vi "Day 7.2 - align crabs subs with increasing fuel cost.vi"(11 "input":i32[](array[numeric])) -> (3 "output":i32)   [LabVIEW 2021]
panel:
  out "position":i32
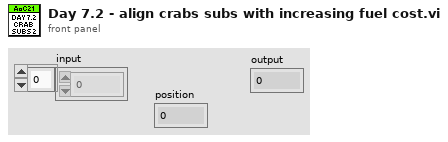
[diagram p1: front panel]
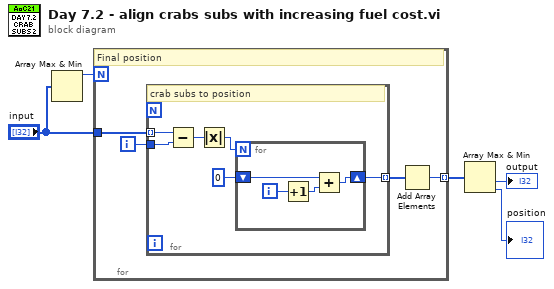
[diagram p0: block diagram]
diagram:
  n1 = Array Max & Min(array="input") -> (max value=w4:i32)  [unwired: 3 out]
  n2 = for {
    N: w4 -> [_]
    tunnel: "input" -> [w9]
    tunnel: [w6] -> w3 mode=indexing
    i -> [w8]
    # "Final position"
    n3 = for {
      tunnel: w8 -> [w14]
      tunnel: w9 -> [w15] mode=indexing
      tunnel: [w10] -> w7 mode=indexing
      # "crab subs to position"
      n4 = Subtract(x=w15, y=w14) -> (x-y=w13:i32)
      n5 = Absolute Value(x=w13) -> (abs(x)=w12:i32)
      n6 = for {
        N: w12 -> [_]
        shift-right: [w16] -> w10
        shift-left: 0 -> [w18]
        i -> [w19]
        n7 = Increment(x=w19) -> (x+1=w17:i32)
        n8 = Add(x=w18, y=w17) -> (x+y=w16:i32)
      }
    }
    n9 = Add Array Elements(numeric array=w7) -> (sum=w6:i32)
  }
  n10 = Array Max & Min(array=w3) -> (min value=→"output":i32, min index (indices)=→"position":i32)  [unwired: 2 out]
